vi "Main.vi"() -> ()   [LabVIEW 2015]
uses:
  <vilib>/Instr/_visa.llb/VISA Configure Serial Port (Instr).vi
panel:
  out "On/Off Set":bool
  out "Measurement History":waveform(dbl)(graph)
  out "Set Point FB":i32 caption="Temp Set Point (C)"
  out "Heater Status":bool
  out "Temp (C)":dbl
  in  "Set Point (C)":i32 caption="Temp Set Point (C)" min=0 max=40
  in  "Heater":bool
  in  "String":string
  in  "Send":bool
  in  "stop":bool
  out "Time of Read":string
  out "Serial Buffer":string
  in  "VISA resource name":refnum<visa-resource-name>
  # "Fluid Heater Control"
  # "Feedback"
  # "Setpoint"
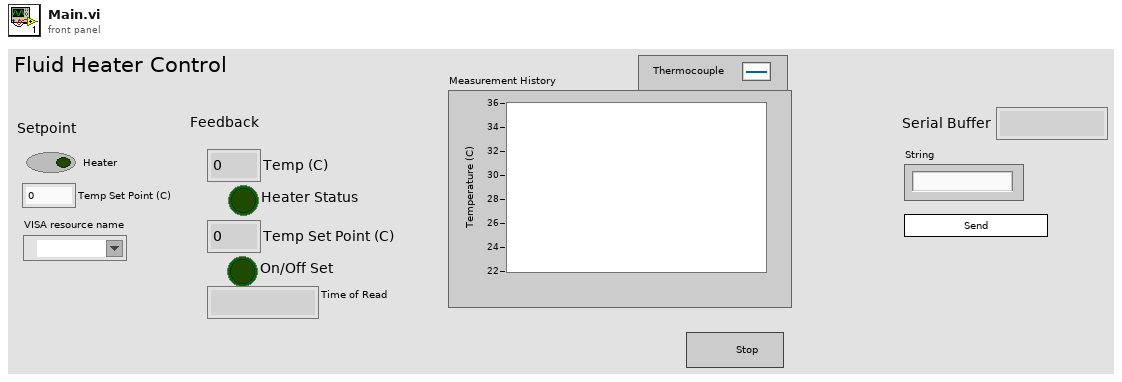
[diagram p1: front panel]
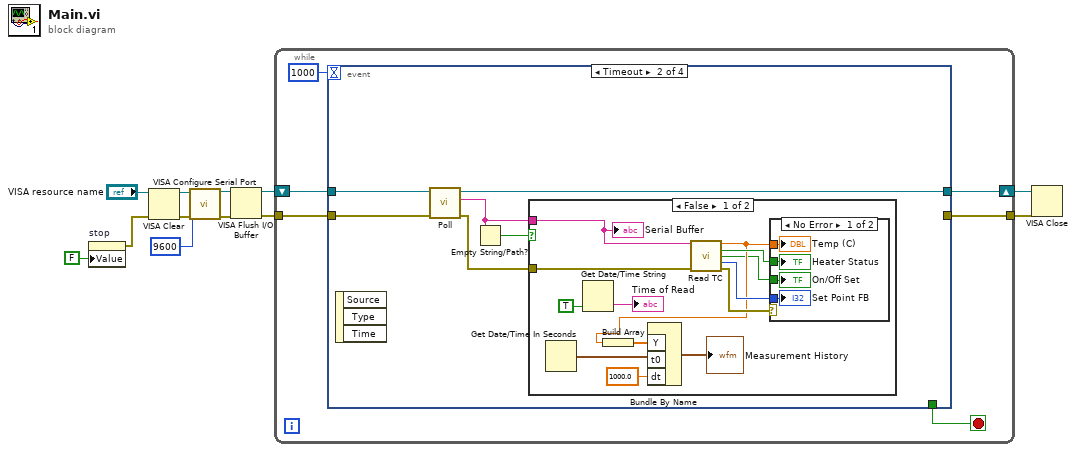
[diagram p0: block diagram]
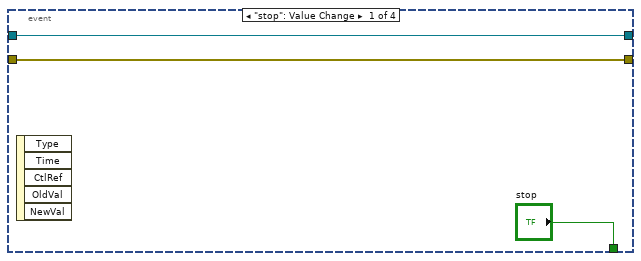
[diagram p2: hidden frame]
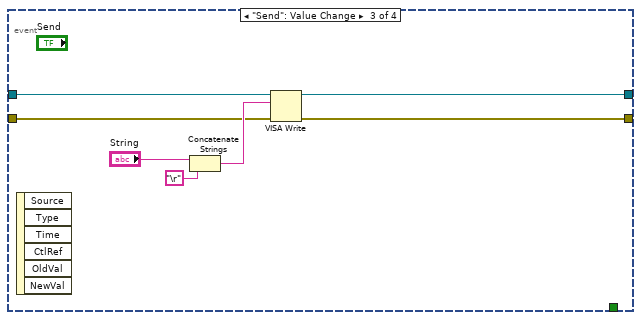
[diagram p5: hidden frame]
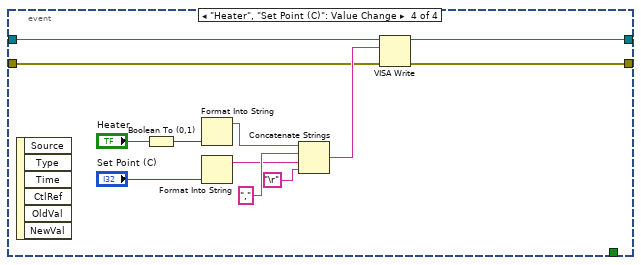
[diagram p6: hidden frame]
diagram:
  n1 = property on="stop" class="Bool (strict)"("Value"=FALSE ("stop")) -> (error out=w2:errorcluster)  [unwired: 2 in, 1 out]
  n2 = VISA Clear(VISA resource name="VISA resource name", error in (no error)=w2) -> (VISA resource name out=w8:refnum<visa-resource-name>, error out=w11:errorcluster)
  n3 = call-poly "VISA Configure Serial Port"("VISA resource name"=w8, "baud rate (9600)"=u32 9600, "error in (no error)"=w11) -> ("VISA resource name out"=w7:refnum<visa-resource-name>, "error out"=w12:errorcluster)  [unwired: 11 in]
  n4 = VISA Flush I/O Buffer(VISA resource name=w7, error in (no error)=w12) -> (VISA resource name out=w6:refnum<visa-resource-name>, error out=w5:errorcluster)  [unwired: 1 in]
  n5 = while {
    tunnel: w5 -> [w15]
    shift-right: [w14] -> w4
    shift-left: w6 -> [w16]
    tunnel: [w13] -> w3
    stop <- w18 stop-if-true
    n6 = event shown="[1] Timeout" {
      selector: _ -> [_ _ _ _]
      dyn-events: _ -> [_ _ _ _]
      timeout: 1000 -> [_ _ _ _]
      tunnel: ["stop" _ _ _] -> w18
      tunnel: w16 -> [w20 w25 w48 w55]
      tunnel: w15 -> [w19 w24 w46 w54]
      tunnel: [w20 w23 w47 w53] -> w14
      tunnel: [w19 _ w45 w52] -> w13
      event "stop": Value Change {
        n7 = event-data() -> ()  [unwired: 1 in, 5 out]
      }
      event Timeout {
        n8 = event-data() -> ()  [unwired: 1 in, 3 out]
        n9 = call "Poll.vi"("error in"=w24, "VISA resource name in"=w25) -> ("error out"=w22:errorcluster, "Read"=w27:string, "VISA resource name out"=w23:refnum<visa-resource-name>)  [unwired: 7 in]
        n10 = Empty String/Path?(string/path=w27) -> (empty?=w26:bool)
        n11 = case shown="False" w26 {
          tunnel: w27 -> [w38 _]
          tunnel: w22 -> [w35 _]
          frame False {
            n12 = Get Date/Time In Seconds() -> (seconds since 1Jan1904=w33:timestamp)
            n13 = Get Date/Time String(want seconds? (F)=TRUE) -> (time string=→"Time of Read":string)  [unwired: 2 in, 1 out]
            n14 = call "Read TC.vi"("read buffer"=w38, "Error In"=w35) -> ("Temp (C)"=w29:dbl, "On/Off Actual"=w37:bool, "On/Off Set"=w28:bool, "Temp Set Point (C)"=w36:i32, "Error Out"=w34:errorcluster)  [unwired: 9 in]
            n15 = Build Array(w29) -> (w32:dbl[])
            n16 = Bundle By Name("Y"=w32, "t0"=w33, "dt"=1000.0) -> (→"Measurement History":waveform(dbl))  [unwired: 1 in]
            n17 = case shown="No Error" w34 {
              tunnel: w29 -> [w44 _]
              tunnel: w37 -> [w43 _]
              tunnel: w36 -> [w42 _]
              tunnel: w28 -> [w41 _]
              frame No Error {
                "Temp (C)" <- w44
                "Heater Status" <- w43
                "Set Point FB" <- w42
                "On/Off Set" <- w41
              }
              frame Error {
              }
            }
            "Serial Buffer" <- w38
          }
          frame True {
          }
        }
      }
      event "Send": Value Change {
        n18 = event-data() -> ()  [unwired: 1 in, 6 out]
        n19 = Concatenate Strings("String", "\r") -> (w49:string)
        n20 = VISA Write(VISA resource name=w48, write buffer=w49, error in (no error)=w46) -> (VISA resource name out=w47:refnum<visa-resource-name>, error out=w45:errorcluster)  [unwired: 1 out]
      }
      event "Heater", "Set Point (C)": Value Change {
        n21 = event-data() -> ()  [unwired: 1 in, 6 out]
        n22 = Boolean To (0,1)(Boolean="Heater") -> (0, 1=w59:i16)
        n23 = Format Into String(w59) -> (resulting string=w56:string)  [unwired: 3 in, 1 out]
        n24 = Format Into String("Set Point (C)") -> (resulting string=w57:string)  [unwired: 3 in, 1 out]
        n25 = Concatenate Strings(w56, ",", w57, "\r") -> (w62:string)
        n26 = VISA Write(VISA resource name=w55, write buffer=w62, error in (no error)=w54) -> (VISA resource name out=w53:refnum<visa-resource-name>, error out=w52:errorcluster)  [unwired: 1 out]
      }
    }
  }
  n27 = VISA Close(VISA resource name=w4, error in (no error)=w3) -> ()  [unwired: 1 out]
